vi "GetHasSubMenu.vi"(8 "error in (no error)":errorcluster, 10 "Item Tags":string[](array[string]), 11 "MenuMap":map{string, T1}(c390)) -> (0 "error out":errorcluster, 3 "HasSubMenu?":bool[](array[boolean]))   [LabVIEW 2021, in "Menu.lvlib" / "Menu.lvclass"]
uses:
  Menu.lvclass
  Menu.lvclass/Menu.ctl
  <vilib>/Utility/miscctls.llb/LVMenuShortCut.ctl
  MenuItems.ctl
  Picture2D/src/Picture/Image.lvclass
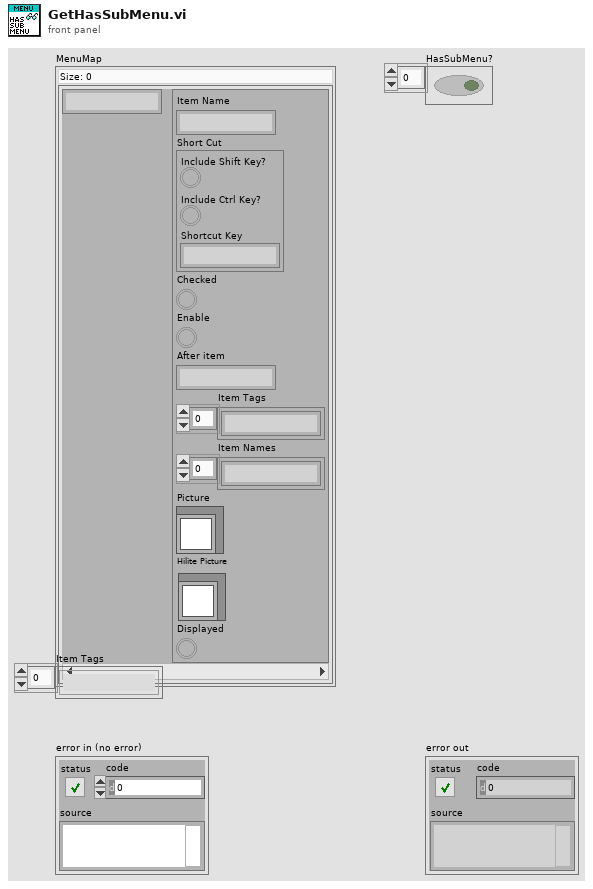
[diagram p1: front panel]
types:
  T1 = typedef "Menu.lvlib/Menu.lvclass/MenuItems.ctl" = cluster{"Item Name":string, "Short Cut":T2, "Checked":bool, "Enable":bool, "After item":string, "Item Tags":string[], "Item Names":string[], "Picture":refnum<class "Image.lvclass">, "Hilite Picture":refnum<class "Image.lvclass">, "Displayed":bool}
  T2 = typedef "LVMenuShortCut.ctl" = cluster{"Include Shift Key?":bool, "Include Ctrl Key?":bool, "Shortcut Key":string}
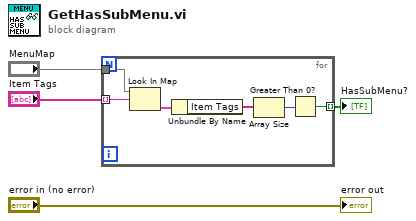
[diagram p0: block diagram]
diagram:
  n1 = for {
    tunnel: "MenuMap" -> [w10]
    tunnel: "Item Tags" -> [w9] mode=indexing
    tunnel: [w5] -> w3 mode=indexing
    n2 = Look In Map(map=w10, key=w9) -> (value=w8:T1)  [unwired: 1 in, 1 out]
    n3 = Unbundle By Name(w8) -> ("Item Tags"=w7:string[])
    n4 = Array Size(array=w7) -> (size(s)=w6:i32)
    n5 = Greater Than 0?(x=w6) -> (x > 0?=w5:bool)
  }
  "HasSubMenu?" <- w3
  "error out" <- "error in (no error)"
